vi "多参数测量数据读取.vi"(8 "Error in":errorcluster caption="Error in (no error)", 11 "探头选择":u16(ring)=9 items=["氨氮"=3, "水温"=9, "pH值"=10, "溶解氧"=11, "电导率"=12, "浊度"=13, "叶绿素a"=14, "藻密度"=15, "蓝绿藻"=16, "氧化还原电位"=17, "溶解氧%"=18, "盐度"=19]) -> (0 "error out":errorcluster, 2 "测量数据块":T1, 3 "添加的数组":string[][](array[string]))   [LabVIEW 2016, in "斯坦道仪器.lvlib"]
panel:
  out "单位":string(combo)
  in  "测量数据区":i32(listbox)
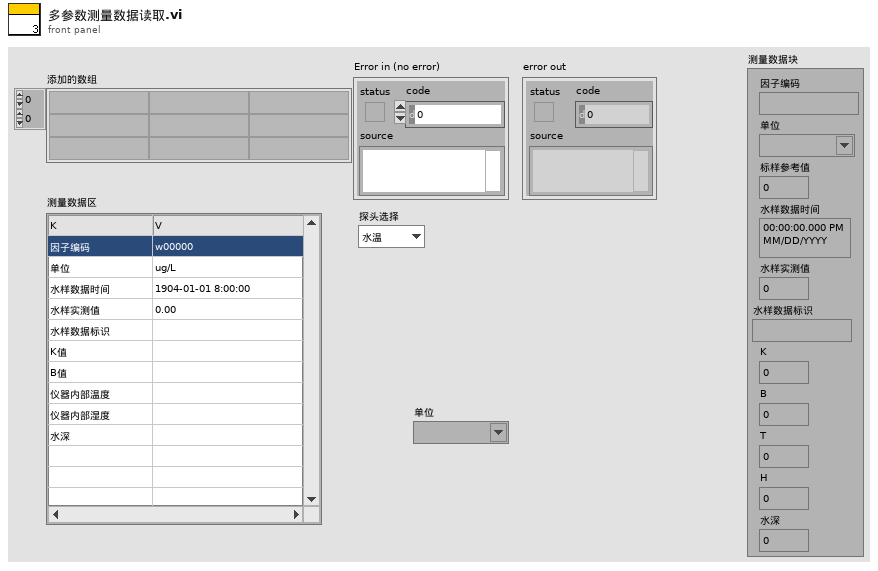
[diagram p1: front panel]
types:
  T1 = cluster{"因子编码":string, "单位":string, "标样参考值":sgl, "水样数据时间":timestamp, "水样实测值":sgl, "水样数据标识":string, "K":sgl, "B":sgl, "T":sgl, "H":sgl, "水深":sgl}
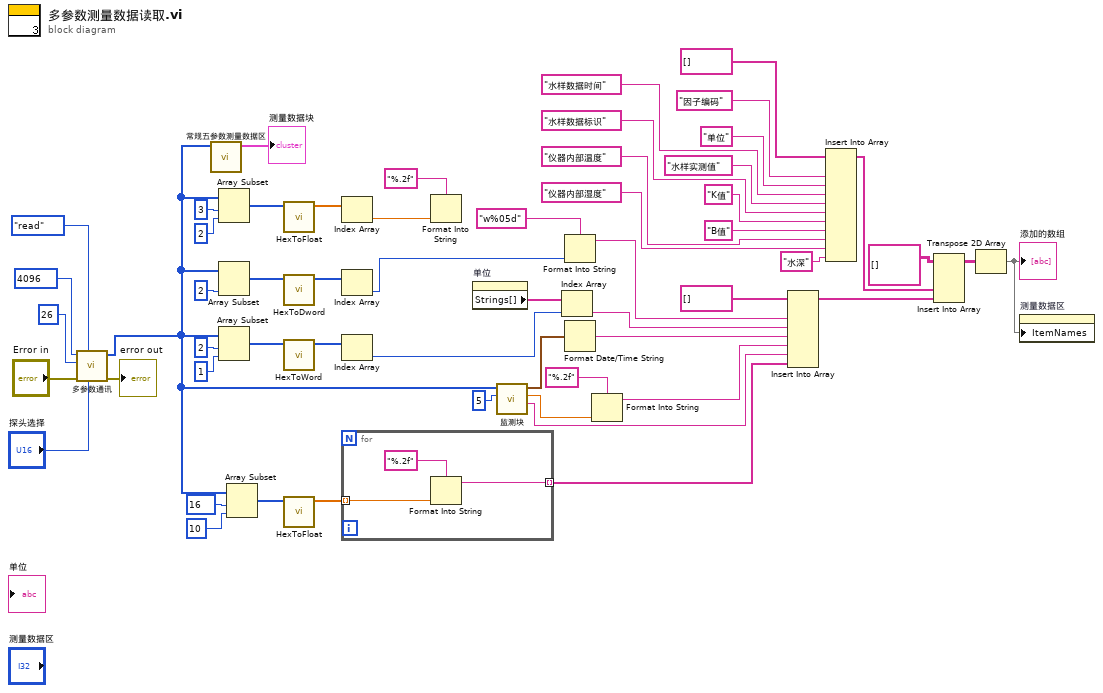
[diagram p0: block diagram]
diagram:
  n1 = call "多参数通讯.vi"("Slave ID"="探头选择", "STEP"=enum16{"open", "read", "write", "close"}."read", "Error in"="Error in", "quantity"=u16 26, "starting address"=u16 4096) -> ("error out"=→"error out":errorcluster, "Registers"=w21:u16[])  [unwired: 4 in, 1 out]
  n2 = call "常规五参数测量数据区.vi"("数组"=w21) -> ("测量数据区"=→"测量数据块":T1)  [unwired: 10 in]
  n3 = Array Subset(array=w21, index=3 ("索引"), length=2 ("长度")) -> (w42:u16[])
  n4 = Array Subset(array=w21, length=2 ("长度")) -> (w51:u16[])  [unwired: 1 in]
  n5 = Array Subset(array=w21, index=2 ("索引"), length=1 ("长度")) -> (w46:u16[])
  n6 = Array Subset(array=w21, index=16 ("索引"), length=10 ("长度")) -> (w37:u16[])
  n7 = call "HexToFloat.vi"("数组"=w42) -> ("FLOAT"=w41:sgl[])  [unwired: 10 in]
  n8 = call "HexToDword.vi"("数组"=w51) -> ("DWORD"=w49:i32[])  [unwired: 10 in]
  n9 = call "HexToWord.vi"("数组"=w46) -> ("WORD"=w45:u16[])  [unwired: 10 in]
  n10 = call "HexToFloat.vi"("数组"=w37) -> ("FLOAT"=w22:sgl[])  [unwired: 10 in]
  n11 = Index Array(array=w41) -> (element=w27:sgl)  [unwired: 1 in]
  n12 = Index Array(array=w49) -> (element=w33:i32)  [unwired: 1 in]
  n13 = Index Array(array=w45) -> (element=w36:u16)  [unwired: 1 in]
  n14 = for {
    tunnel: w22 -> [w58] mode=indexing
    tunnel: [w57] -> w23 mode=indexing
    n15 = Format Into String(format string="%.2f" ("格式字符串"), w58) -> (resulting string=w57:string)  [unwired: 2 in, 1 out]
  }
  n16 = Format Into String(format string="%.2f" ("格式字符串"), w27) -> ()  [unwired: 2 in, 2 out]
  n17 = property on="单位" class="CmbBox"() -> ("Strings[]"=w35:string[])  [unwired: 2 in, 2 out]
  n18 = call "监测块.vi"("索引"=5, "数组"=w21) -> ("string"=w24:string, "数值"=w30:sgl, "time stamp"=w32:timestamp)  [unwired: 7 in]
  n19 = Index Array(array=w35, index=w36) -> (element=w19:string)
  n20 = Format Into String(format string="w%05d" ("格式字符串"), w33) -> (resulting string=w18:string)  [unwired: 2 in, 1 out]
  n21 = Format Date/Time String(seconds (now)=w32) -> (date/time string=w26:string)  [unwired: 2 in]
  n22 = Format Into String(format string="%.2f" ("格式字符串"), w30) -> (resulting string=w25:string)  [unwired: 2 in, 1 out]
  n23 = Insert Into Array(array=string[] [] ("数组"), new element #1=w18, new element #2=w19, new element #3=w26, new element #4=w25, new element #5=w24, new element #6=w23) -> (w5:string[])  [unwired: 1 in]
  n24 = Insert Into Array(array=string[] [], new element #1="因子编码", new element #2="单位", new element #3="水样数据时间", new element #4="水样实测值", new element #5="水样数据标识", new element #6="K值", new element #7="B值", new element #8="仪器内部温度", new element #9="仪器内部湿度", new element #10="水深") -> (w6:string[])  [unwired: 1 in]
  n25 = Insert Into Array(array=string[][] [], new element #1=w6, new element #2=w5) -> (w4:string[][])  [unwired: 2 in]
  n26 = Transpose 2D Array(2D array=w4) -> (transposed array=w54:string[][])
  "添加的数组" <- w54
  n27 = property on="测量数据区" class="MCListbox (严格)"("ItemNames"=w54) -> ()  [unwired: 2 in, 2 out]
